vi "Insert Bus Monitor.vi"(8 "error in (no error)":errorcluster, 10 "Protected Subpanel":T1, 11 "Mediator in":refnum<class "Mediator.lvclass">) -> (0 "error out":errorcluster, 3 "Mediator out":refnum<class "Mediator.lvclass">)   [LabVIEW 2015, in "Mediator.lvlib" / "Mediator.lvclass"]
uses:
  Mediator.lvclass
  IViewable/ProtectedSubpanel/Protected Subpanel Reference.ctl
  IViewable/ProtectedSubpanel/ProtectedSubpanel.lvclass
  Mediator.lvclass/Mediator.ctl
  IViewable/IViewable Messages/Insert View Msg/Insert View Msg.lvclass/Insert View Msg.ctl
  <vilib>/ActorFramework/Message Enqueuer/Message Enqueuer.lvclass/Message Enqueuer.ctl
  <vilib>/ActorFramework/Message Enqueuer/Enqueue.vi
  <vilib>/ActorFramework/Message Priority Queue/Priority Enqueue.vi
  <vilib>/ActorFramework/Message Enqueuer/Message Enqueuer.lvclass
  IViewable/IViewable Messages/Insert View Msg/Insert View Msg.lvclass
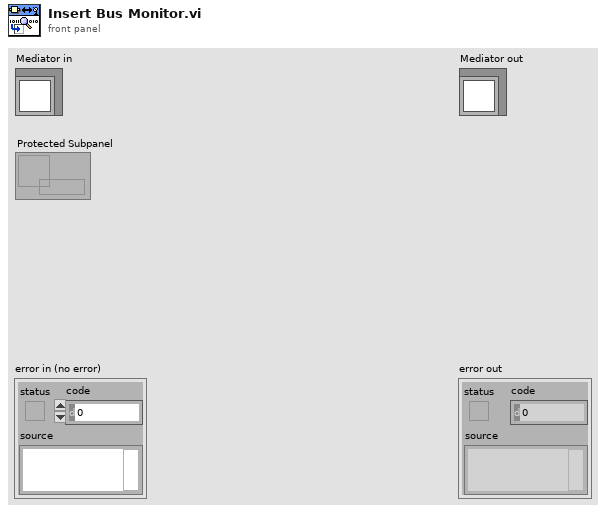
[diagram p1: front panel]
types:
  T1 = typedef "IViewable.lvlib/ProtectedSubpanel.lvclass/Protected Subpanel Reference.ctl" = refnum<data-value>
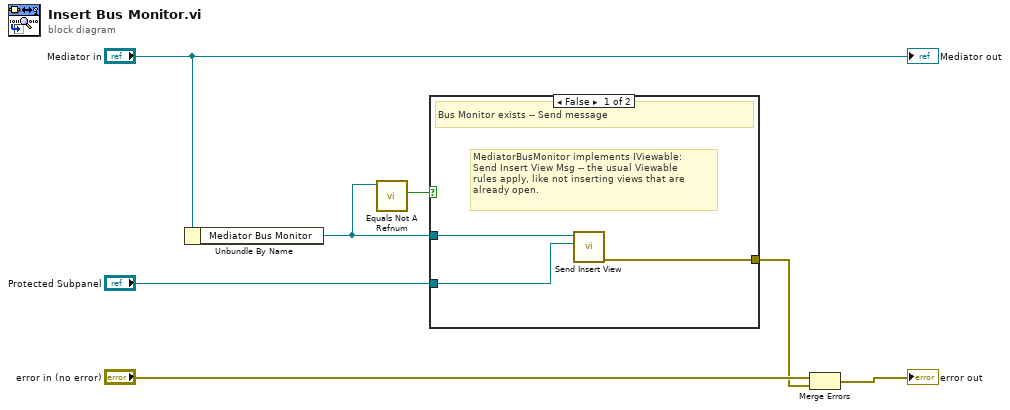
[diagram p0: block diagram]
diagram:
  n1 = Unbundle By Name("Mediator in") -> ("Mediator Bus Monitor"=w2:refnum<class "Message Enqueuer.lvclass">)
  n2 = call <vilib>:"Equals Not A Refnum.vi"("Message Enqueuer"=w2) -> ("Not a refnum?"=w1:bool)  [unwired: 10 in]
  n3 = case shown="False" w1 {
    tunnel: w2 -> [w10 _]
    tunnel: "Protected Subpanel" -> [w9 _]
    tunnel: [w8 _] -> w3
    frame False {
      # "MediatorBusMonitor implements IViewable:\nSend Insert View Msg -- the usual Viewable\nrules apply, like not inserting views that are\nalready open."
      # "Bus Monitor exists -- Send message"
      n4 = call "Send Insert View.vi"("Protected Subpanel"=w9, "Message Enqueuer"=w10) -> ("error out"=w8:errorcluster)  [unwired: 8 in, 1 out]
    }
    frame True {
      # "No Bus Monitor -- Send nothing"
    }
  }
  n5 = Merge Errors("error in (no error)", w3) -> (→"error out":errorcluster)
  "Mediator out" <- "Mediator in"
